vi "GlobalErrorIndex.vi"() -> ()   [LabVIEW 2015]
panel:
  out "Err Index":dbl
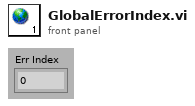
[diagram p1: front panel]
diagram:
